vi "FRCts20_WebMethods_GetSessionInfo.vi"(8 "error in":errorcluster, 11 "httpRequestID":u32) -> (0 "error out":errorcluster, 2 "Return Type":T1="mobile", 3 "httpRequestID out":u32)   [LabVIEW 2014, in "FRCts20_WebMethods.lvlib"]
doc: "Extracts the <B>Accept</B> and <B>User-Agent</B> HTTP Request variables to determine the type of content to return to the client.\n\nPossible return types: plain (text), xml, mobile (html), desktop (html)\n\n<B>Accept</B> variable overrides <B>User-Agent</B>."
uses:
  FRCts20_WebMethods.lvlib
  Controls/FRCts20_WebMethods_ctl_returntype.ctl
  <vilib>/regexp/Match Regular Expression.xnode
  <vilib>/wsapi/NI_WebServices.lvlib
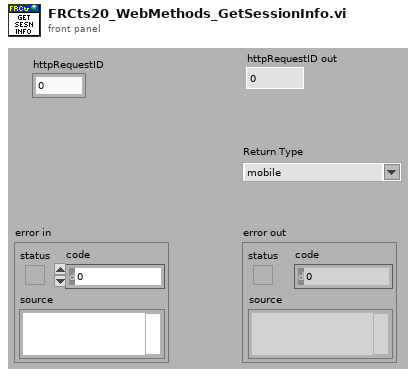
[diagram p1: front panel]
types:
  T1 = typedef "FRCts20_WebMethods.lvlib/FRCts20_WebMethods_ctl_returntype.ctl" = string
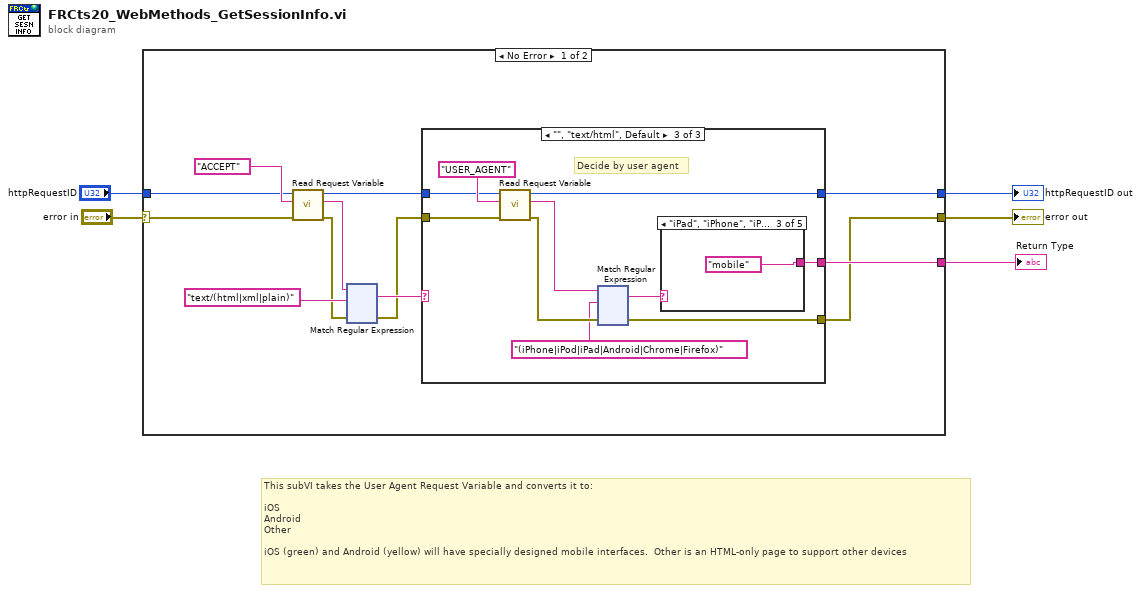
[diagram p0: block diagram]
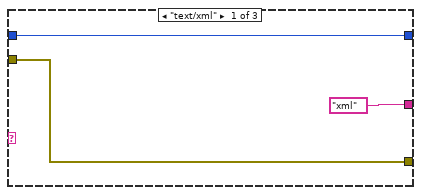
[diagram p2: hidden frame]
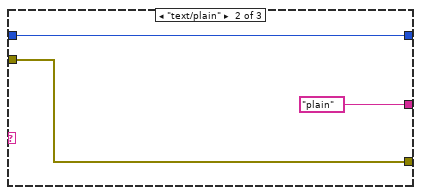
[diagram p3: hidden frame]
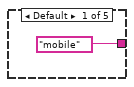
[diagram p4: hidden frame]
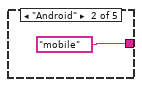
[diagram p5: hidden frame]
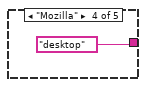
[diagram p6: hidden frame]
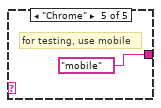
[diagram p7: hidden frame]
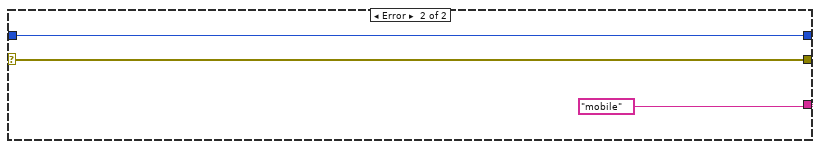
[diagram p8: hidden frame]
diagram:
  # "This subVI takes the User Agent Request Variable and converts it to:\n\niOS\nAndroid\nOther\n\niOS (green) and Android (yellow) will have specially designed mobile interfaces.  Other is an HTML-only page to support other devices"
  n1 = case shown="No Error" "error in" {
    selector: "error in" -> [w9 w263]
    tunnel: [w6 w263] -> w4
    tunnel: "httpRequestID" -> [w8 w262]
    tunnel: [w7 w262] -> w2
    tunnel: [w17 T1 "mobile" ("Return")] -> w1
    frame No Error {
      n2 = call <vilib>:"Read Request Variable.vi"("error in (no error)"=w9, "variable name"="ACCEPT", "httpRequestID"=w8) -> ("error out"=w13:errorcluster, "value"=w15:string, "httpRequestID out"=w11:u32)  [unwired: 6 in]
      n3 = xnode "Match Regular Expression"("input string"=w15, "regular expression"="text/(html|xml|plain)", "error in"=w13) -> ("whole match"=w12:string, "error out"=w10:errorcluster)  [unwired: 3 in, 3 out]
      n4 = case shown="\"\", \"text/html\", Default" w12 {
        tunnel: w11 -> [w129 w134 w139]
        tunnel: w10 -> [w130 w133 w138]
        tunnel: [w130 w133 w137] -> w6
        tunnel: [w129 w134 w136] -> w7
        tunnel: [T1 "xml" ("Return") T1 "plain" ("Return") w135] -> w17
        frame "text/xml" {
        }
        frame "text/plain" {
        }
        frame "", "text/html", Default {
          # "Decide by user agent"
          n5 = call <vilib>:"Read Request Variable.vi"("error in (no error)"=w138, "variable name"="USER_AGENT", "httpRequestID"=w139) -> ("error out"=w144:errorcluster, "value"=w143:string, "httpRequestID out"=w136:u32)  [unwired: 6 in]
          n6 = xnode "Match Regular Expression"("input string"=w143, "regular expression"="(iPhone|iPod|iPad|Android|Chrome|Firefox)", "error in"=w144) -> ("whole match"=w142:string, "error out"=w137:errorcluster)  [unwired: 3 in, 3 out]
          n7 = case shown="\"iPad\", \"iPhone\", \"iPod\"" w142 {
            tunnel: [T1 "mobile" ("Return") T1 "mobile" ("Return") T1 "mobile" ("Return") T1 "desktop" ("Return") T1 "mobile" ("Return")] -> w135
            frame Default {
            }
            frame "Android" {
            }
            frame "iPad", "iPhone", "iPod" {
            }
            frame "Mozilla" {
            }
            frame "Chrome" {
              # "for testing, use mobile"
            }
          }
        }
      }
    }
    frame Error {
    }
  }
  "error out" <- w4
  "httpRequestID out" <- w2
  "Return Type" <- w1
